vi "DSF Config File to Engine Config Cluster.vi"(8 "error in (no error)":errorcluster, 10 "engine offsets":u64[](array[numeric]), 11 "dsf configuration file path":path) -> (0 "error out":errorcluster, 3 "output cluster":T1)   [LabVIEW 2017, in "DSF.Engine.lvlib"]
uses:
  DSF.Engine.lvlib
  DSF Configuration API/1.0.0/Public/Controls/DSF Engine Framework Configuration.ctl
  DSF Configuration API/1.0.0/Public/Controls/DSF Engine Plugin Configuration.ctl
  DSF Configuration API/1.0.0/Public/Controls/DSF Timing Info.ctl
  DSF Configuration API/1.0.0/Public/Controls/DSF Engine Transfer Group Configuration.ctl
  DSF Configuration API/1.0.0/Public/Controls/DSF Direction.ctl
  DSF Configuration API/1.0.0/Public/Controls/DSF Engine Transfer Configuration.ctl
  DSF Configuration API/1.0.0/Public/Controls/DSF Byte Order.ctl
  DSF Configuration API/1.0.0/Public/Controls/DSF Engine Channel Configuration.ctl
  DSF Configuration API/1.0.0/Public/Controls/DSF Data Type.ctl
  DSF Configuration API/1.0.0/Public/Controls/DSF Settings Info.ctl
  DSF Configuration API/1.0.0/Public/Read All Item IDs/Read All Plugin IDs.vi
  DSF Configuration API/1.0.0/Public/Read Item/Read Plugin.vi
  DSF Configuration API/1.0.0/Public/Read Item/Read Settings.vi
  DSF Configuration API/1.0.0/Public/Read Item/Read Group.vi
  DSF Configuration API/1.0.0/Public/Read Item/Read Transfer.vi
  DSF Configuration API/1.0.0/Public/Read Item/Read Channel.vi
  DSF Configuration API/1.0.0/DSF Configuration API.lvlib
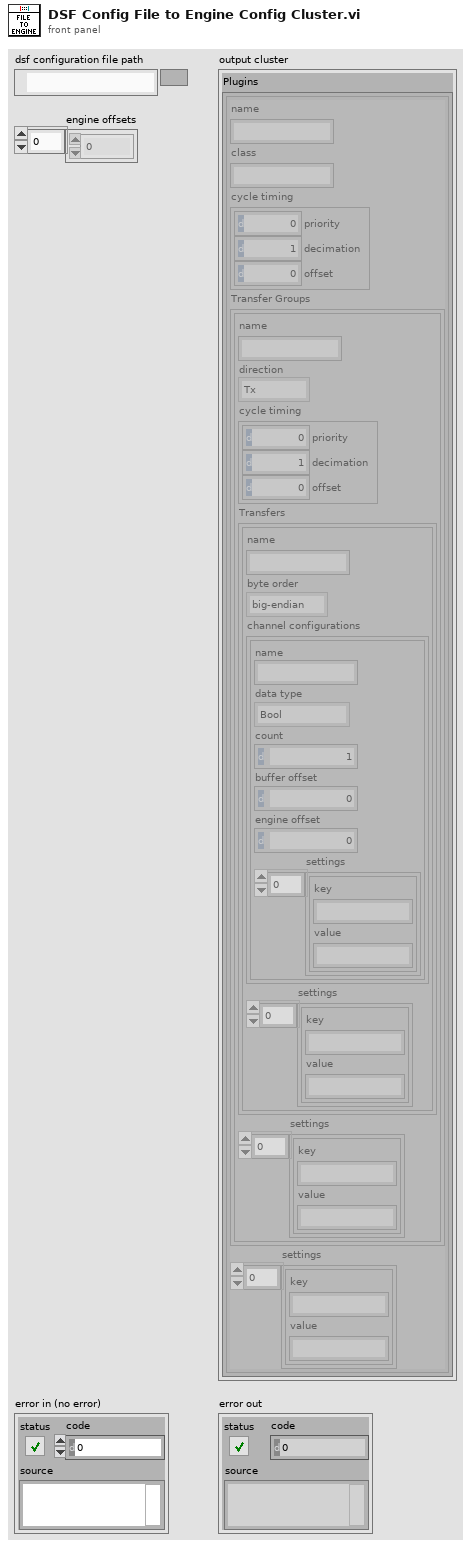
[diagram p1: front panel]
types:
  T1 = typedef "DSF Configuration API.lvlib/DSF Engine Framework Configuration.ctl" = cluster{"Plugins":T2[]}
  T2 = typedef "DSF Configuration API.lvlib/DSF Engine Plugin Configuration.ctl" = cluster{"name":string, "class":string, "cycle timing":T3, "Transfer Groups":T4[], "settings":T10}
  T3 = typedef "DSF Configuration API.lvlib/DSF Timing Info.ctl" = cluster{"priority":i32, "decimation":i32, "offset":i32}
  T4 = typedef "DSF Configuration API.lvlib/DSF Engine Transfer Group Configuration.ctl" = cluster{"name":string, "direction":T5, "cycle timing":T3, "Transfers":T6[], "settings":T10}
  T5 = typedef "DSF Configuration API.lvlib/DSF Direction.ctl" = enum8{"Tx", "Rx"}
  T6 = typedef "DSF Configuration API.lvlib/DSF Engine Transfer Configuration.ctl" = cluster{"name":string, "byte order":T7, "channel configurations":T8[], "settings":T10}
  T7 = typedef "DSF Configuration API.lvlib/DSF Byte Order.ctl" = enum8{"big-endian", "little-endian"}
  T8 = typedef "DSF Configuration API.lvlib/DSF Engine Channel Configuration.ctl" = cluster{"name":string, "data type":T9, "count":u64, "buffer offset":u64, "engine offset":u64, "settings":T10}
  T9 = typedef "DSF Configuration API.lvlib/DSF Data Type.ctl" = enum8{"Bool", "SGL", "DBL", "I8", "I16", "I32", "I64", "U8", "U16", "U32", "U64"}
  T10 = typedef "DSF Configuration API.lvlib/DSF Settings Info.ctl" = cluster{"key":string, "value":string}[]
  T11 = typedef "DSF Configuration API.lvlib/DSF Config Data RefNum.ctl" = refnum<k1>
  T12 = typedef "DSF Configuration API.lvlib/DSF Plugin Info.ctl" = cluster{"type":string, "timing":T3, "group ids":string[], "settings id":string}
  T13 = typedef "DSF Configuration API.lvlib/DSF Group Info.ctl" = cluster{"direction":T5, "timing":T3, "transfer ids":string[], "settings id":string}
  T14 = typedef "DSF Configuration API.lvlib/DSF Transfer Info.ctl" = cluster{"byte order":T7, "channel ids":string[], "settings id":string}
  T15 = typedef "DSF Configuration API.lvlib/DSF Channel Info.ctl" = cluster{"count":u64, "buffer offset":u64, "engine offset":u64, "data type":T9, "settings id":string}
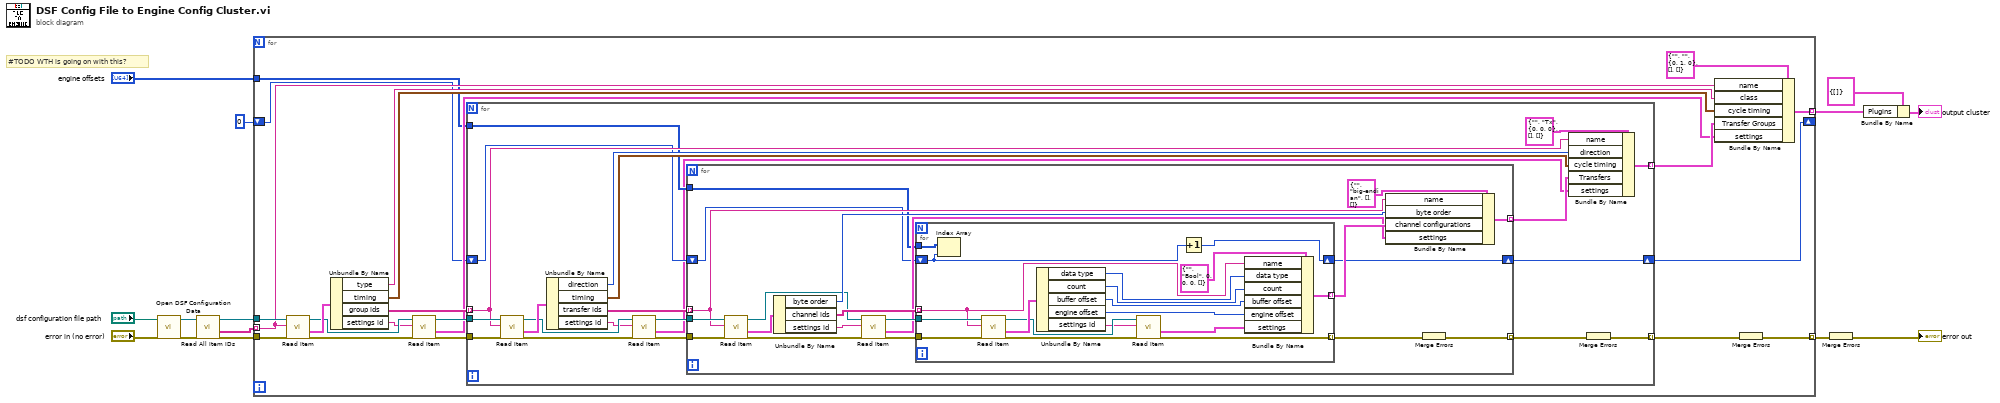
[diagram p0: block diagram]
diagram:
  # "#TODO WTH is going on with this?"
  n1 = call "Open DSF Configuration Data.vi"("error in (no error)"="error in (no error)", "dsf configuration file path"="dsf configuration file path") -> ("error out"=w11:errorcluster, "dsf refnum"=w12:T11)  [unwired: 5 in, 3 out]
  n2 = call-poly "Read All Item IDs.vi"("error in (no error)"=w11, "dsf refnum"=w12) -> ("error out"=w7:errorcluster, "Plugin IDs"=w9:string[], "dsf refnum out"=w8:T11)  [unwired: 7 in]
  n3 = for {
    tunnel: w9 -> [w27] mode=indexing
    tunnel: w8 -> [w34]
    tunnel: [w30] -> w1 mode=indexing
    tunnel: w7 -> [w21]
    tunnel: "engine offsets" -> [w19]
    shift-right: [w17] -> _
    shift-left: 0 -> [w18]
    tunnel: [w15] -> w4 mode=indexing
    n4 = call-poly "Read Item.vi"("error in (no error)"=w21, "Plugin ID"=w27, "dsf refnum"=w34) -> ("error out"=w22:errorcluster, "value"=w33:T12, "dsf refnum out"=w26:T11)  [unwired: 5 in, 1 out]
    n5 = Unbundle By Name(w33) -> ("type"=w32:string, "timing"=w31:T3, "group ids"=w29:string[], "settings id"=w24:string)
    n6 = call-poly "Read Item.vi"("error in (no error)"=w22, "Settings ID"=w24, "dsf refnum"=w26) -> ("error out"=w20:errorcluster, "value"=w23:T10, "dsf refnum out"=w25:T11)  [unwired: 5 in, 1 out]
    n7 = for {
      tunnel: w25 -> [w56]
      tunnel: w29 -> [w53] mode=indexing
      tunnel: [w50] -> w28 mode=indexing
      tunnel: w20 -> [w47]
      tunnel: w19 -> [w41]
      shift-right: [w39] -> w17
      shift-left: w18 -> [w40]
      tunnel: [w36] -> w16 mode=indexing
      n8 = call-poly "Read Item.vi"("error in (no error)"=w47, "Group ID"=w53, "dsf refnum"=w56) -> ("error out"=w43:errorcluster, "value"=w54:T13, "dsf refnum out"=w46:T11)  [unwired: 5 in, 1 out]
      n9 = Unbundle By Name(w54) -> ("direction"=w52:T5, "timing"=w51:T3, "transfer ids"=w49:string[], "settings id"=w44:string)
      n10 = call-poly "Read Item.vi"("error in (no error)"=w43, "Settings ID"=w44, "dsf refnum"=w46) -> ("error out"=w42:errorcluster, "value"=w38:T10, "dsf refnum out"=w45:T11)  [unwired: 5 in, 1 out]
      n11 = for {
        tunnel: w49 -> [w69] mode=indexing
        tunnel: w45 -> [w76]
        tunnel: [w73] -> w48 mode=indexing
        tunnel: w42 -> [w68]
        tunnel: w41 -> [w62]
        shift-right: [w60] -> w39
        shift-left: w40 -> [w61]
        tunnel: [w58] -> w37 mode=indexing
        n12 = call-poly "Read Item.vi"("error in (no error)"=w68, "Transfer ID"=w69, "dsf refnum"=w76) -> ("error out"=w66:errorcluster, "value"=w75:T14, "dsf refnum out"=w70:T11)  [unwired: 5 in, 1 out]
        n13 = Unbundle By Name(w75) -> ("byte order"=w74:T7, "channel ids"=w71:string[], "settings id"=w65:string)
        n14 = call-poly "Read Item.vi"("error in (no error)"=w66, "Settings ID"=w65, "dsf refnum"=w70) -> ("error out"=w64:errorcluster, "value"=w63:T10, "dsf refnum out"=w67:T11)  [unwired: 5 in, 1 out]
        n15 = for {
          tunnel: [w94] -> w72 mode=indexing
          tunnel: w71 -> [w92] mode=indexing
          tunnel: w67 -> [w93]
          tunnel: w64 -> [w87]
          tunnel: w62 -> [w82]
          shift-right: [w81] -> w60
          shift-left: w61 -> [w78]
          tunnel: [w80] -> w59 mode=indexing
          n16 = Index Array(array=w82, index=w78) -> ()  [unwired: 1 out]
          n17 = call-poly "Read Item.vi"("error in (no error)"=w87, "Channel ID"=w92, "dsf refnum"=w93) -> ("error out"=w85:errorcluster, "value"=w91:T15, "dsf refnum out"=w86:T11)  [unwired: 5 in, 1 out]
          n18 = Unbundle By Name(w91) -> ("data type"=w90:T9, "count"=w89:u64, "buffer offset"=w88:u64, "engine offset"=w77:u64, "settings id"=w84:string)
          n19 = call-poly "Read Item.vi"("error in (no error)"=w85, "Settings ID"=w84, "dsf refnum"=w86) -> ("error out"=w80:errorcluster, "value"=w83:T10)  [unwired: 5 in, 2 out]
          n20 = Increment(x=w78) -> (x+1=w81:i32)
          n21 = Bundle By Name(cluster=T8 {"name"="", "data type"=enum."Bool", "count"=0, "buffer offset"=0, "engine offset"=0, "settings"=[]} ("channel configurations"), "name"=w92, "data type"=w90, "count"=w89, "buffer offset"=w88, "engine offset"=w77, "settings"=w83) -> (w94:T8)
        }
        n22 = Bundle By Name(cluster=T6 {"name"="", "byte order"=enum."big-endian", "channel configurations"=[], "settings"=[]} ("Transfer Configuration"), "name"=w69, "byte order"=w74, "channel configurations"=w72, "settings"=w63) -> (w73:T6)
        n23 = Merge Errors(w59) -> (w58:errorcluster)
      }
      n24 = Bundle By Name(cluster=T4 {"name"="", "direction"=enum."Tx", "cycle timing"={"priority"=0, "decimation"=0, "offset"=0}, "Transfers"=[], "settings"=[]} ("Transfer Group Configuration"), "name"=w53, "direction"=w52, "cycle timing"=w51, "Transfers"=w48, "settings"=w38) -> (w50:T4)
      n25 = Merge Errors(w37) -> (w36:errorcluster)
    }
    n26 = Bundle By Name(cluster=T2 {"name"="", "class"="", "cycle timing"={"priority"=0, "decimation"=1, "offset"=0}, "Transfer Groups"=[], "settings"=[]} ("Plugin Configuration"), "name"=w27, "class"=w32, "cycle timing"=w31, "Transfer Groups"=w28, "settings"=w23) -> (w30:T2)
    n27 = Merge Errors(w16) -> (w15:errorcluster)
  }
  n28 = Merge Errors(w4) -> (→"error out":errorcluster)
  n29 = Bundle By Name(cluster=T1 {"Plugins"=[]} ("Framework Config (JSON)"), "Plugins"=w1) -> (→"output cluster":T1)
